vi "lj_test_analog_only.vi"(6 "Period [ms]":i32=500 min=1 max=60000) -> (0 "error out":errorcluster)   [LabVIEW 2025, in "LabJackEKG.lvlib"]
uses:
  LabJackEKG.lvlib
panel:
  out "Waveform Chart":i32[](graph)
  in  "Sampling Frequency [Hz]":dbl format="%_2f"
  in  "RSI":i32
  out "Waveform Graph":dbl[][](graph)
  in  "stop":bool
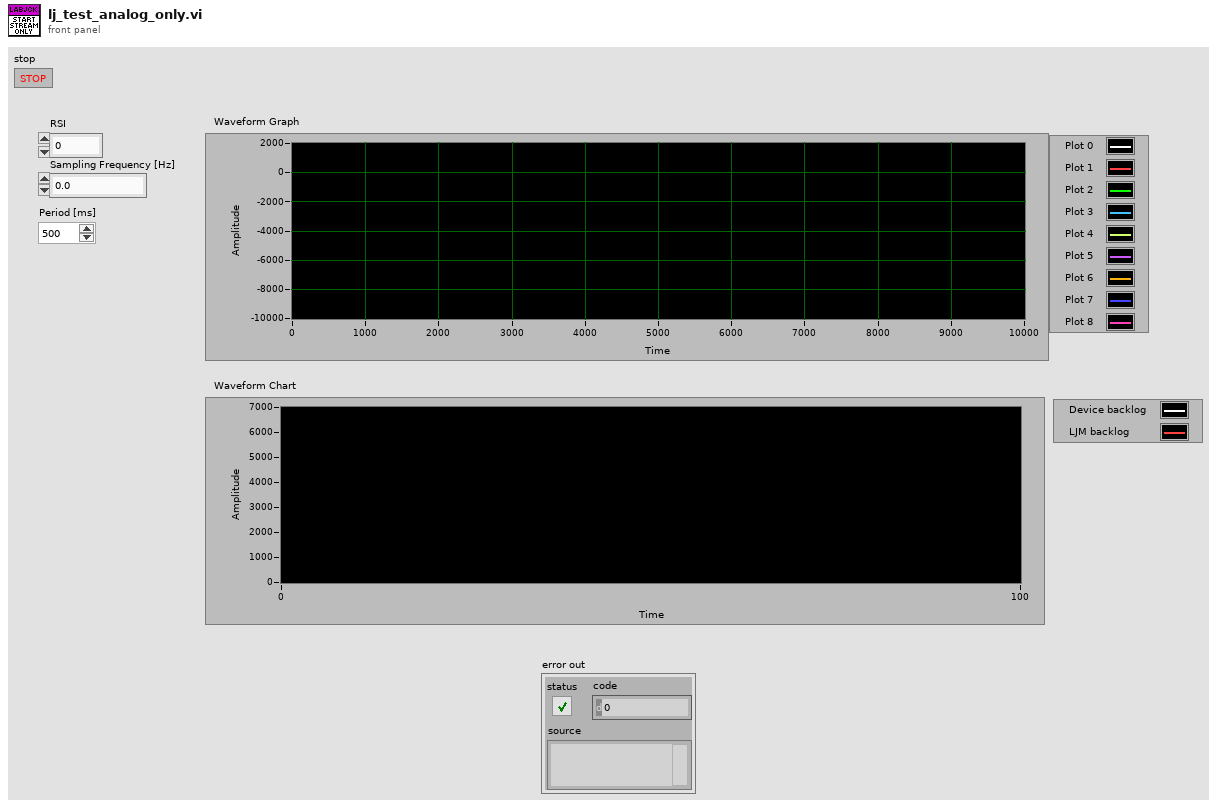
[diagram p1: front panel]
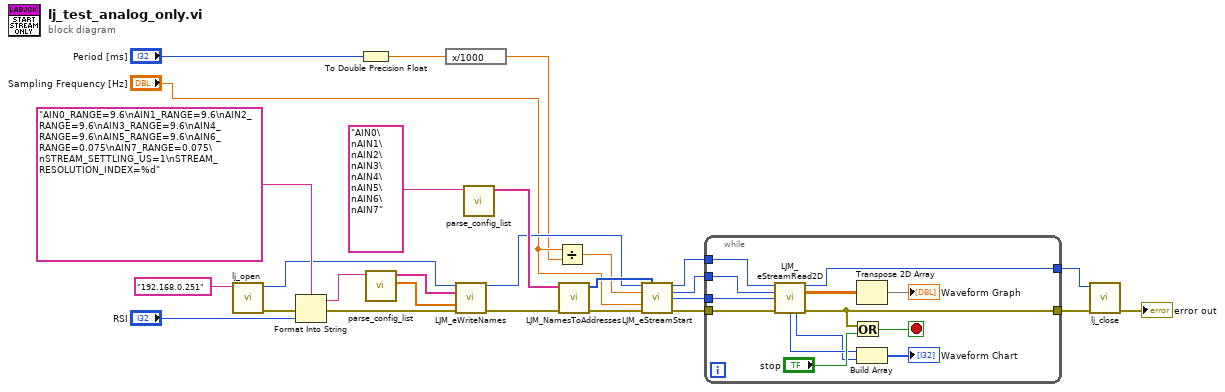
[diagram p0: block diagram]
diagram:
  n1 = call "lj_open.vi"("IP Address (LJM_idANY )"="192.168.0.251") -> ("error out"=w14:errorcluster, "Handle"=w15:i32)  [unwired: 8 in, 1 out]
  n2 = Format Into String(format string="AIN0_RANGE=9.6\nAIN1_RANGE=9.6\nAIN2_RANGE=9.6\nAIN3_RANGE=9.6\nAIN4_RANGE=9.6\nAIN5_RANGE=9.6\nAIN6_RANGE=0.075\nAIN7_RANGE=0.075\nSTREAM_SETTLING_US=1\nSTREAM_RESOLUTION_INDEX=%d" ("String"), error in=w14, "RSI") -> (resulting string=w17:string, error out=w19:errorcluster)  [unwired: 1 in]
  n3 = To Double Precision Float(number="Period [ms]") -> (double precision float=w1:dbl)
  n4 = call "parse_config_list.vi"("String"=w17) -> ("Values"=w26:dbl[], "Names"=w27:string[])  [unwired: 9 in]
  n5 = expression code="x/1000"(w1) -> (w2:dbl)
  n6 = call <vilib>:"LJM_eWriteNames.vi"("Handle In"=w15, "aNames"=w27, "aValuesIn"=w26, "error in"=w19) -> ("Handle Out"=w20:i32, "error out"=w21:errorcluster)  [unwired: 9 in, 1 out]
  n7 = call "parse_config_list.vi"("String"="AIN0\nAIN1\nAIN2\nAIN3\nAIN4\nAIN5\nAIN6\nAIN7") -> ("Names"=w24:string[])  [unwired: 9 in, 1 out]
  n8 = Divide(x="Sampling Frequency [Hz]", y=w2) -> (x/y=w5:dbl)
  n9 = call <vilib>:"LJM_NamesToAddresses.vi"("error in"=w21, "aNames"=w24) -> ("error out"=w22:errorcluster, "aAddresses"=w23:i32[])  [unwired: 7 in, 1 out]
  n10 = call <vilib>:"LJM_eStreamStart.vi"("Handle In"=w20, "aScanList"=w23, "ScansPerRead"=w5, "ScanRate"="Sampling Frequency [Hz]", "error in"=w22) -> ("Handle Out"=w9:i32, "ScansPerRead Out"=w10:i32, "NumReadAddresses"=w11:i32, "error out"=w13:errorcluster)  [unwired: 5 in, 2 out]
  n11 = while {
    tunnel: w13 -> [w40]
    tunnel: [w33] -> w12
    tunnel: w11 -> [w38]
    tunnel: w10 -> [w37]
    tunnel: w9 -> [w36]
    tunnel: [w31] -> w7
    stop <- w34 stop-if-true
    n12 = call <vilib>:"LJM_eStreamRead2D.vi"("Handle In"=w36, "ScansPerRead"=w37, "NumAddresses"=w38, "error in"=w40) -> ("Handle Out"=w31:i32, "aData Out"=w35:dbl[][], "DeviceScanBacklog"=w30:i32, "LJMScanBacklog"=w29:i32, "error out"=w33:errorcluster)  [unwired: 7 in]
    n13 = Or(x=w33, y="stop") -> (x .or. y?=w34:bool)
    n14 = Transpose 2D Array(2D array=w35) -> (transposed array=→"Waveform Graph":dbl[][])
    n15 = Build Array(w30, w29) -> (→"Waveform Chart":i32[])
  }
  n16 = call "lj_close.vi"("error in"=w12, "Handle"=w7) -> ("error out"=→"error out":errorcluster)  [unwired: 9 in]
